vi "Check and Create Kalman Data.vi"(8 "Variance Memory":i32=1, 9 "R":T1, 10 "Pk":T1, 11 "x_k":T1) -> (1 "R out":T1, 2 "Pk out":T1, 3 "x_k out":T1)   [LabVIEW 2018]
uses:
  <vilib>/Analysis/Matrix/Datatypes/RealMatrix.ctl
  <vilib>/Analysis/Matrix/Numeric/Conversions/Array To Matrix - RA2.vi
  <vilib>/Analysis/7linalg.llb/Create Special Real Matrix.vi
  <vilib>/Analysis/Matrix/NI_Matrix.lvlib
  <vilib>/Analysis/NI_AALPro.lvlib
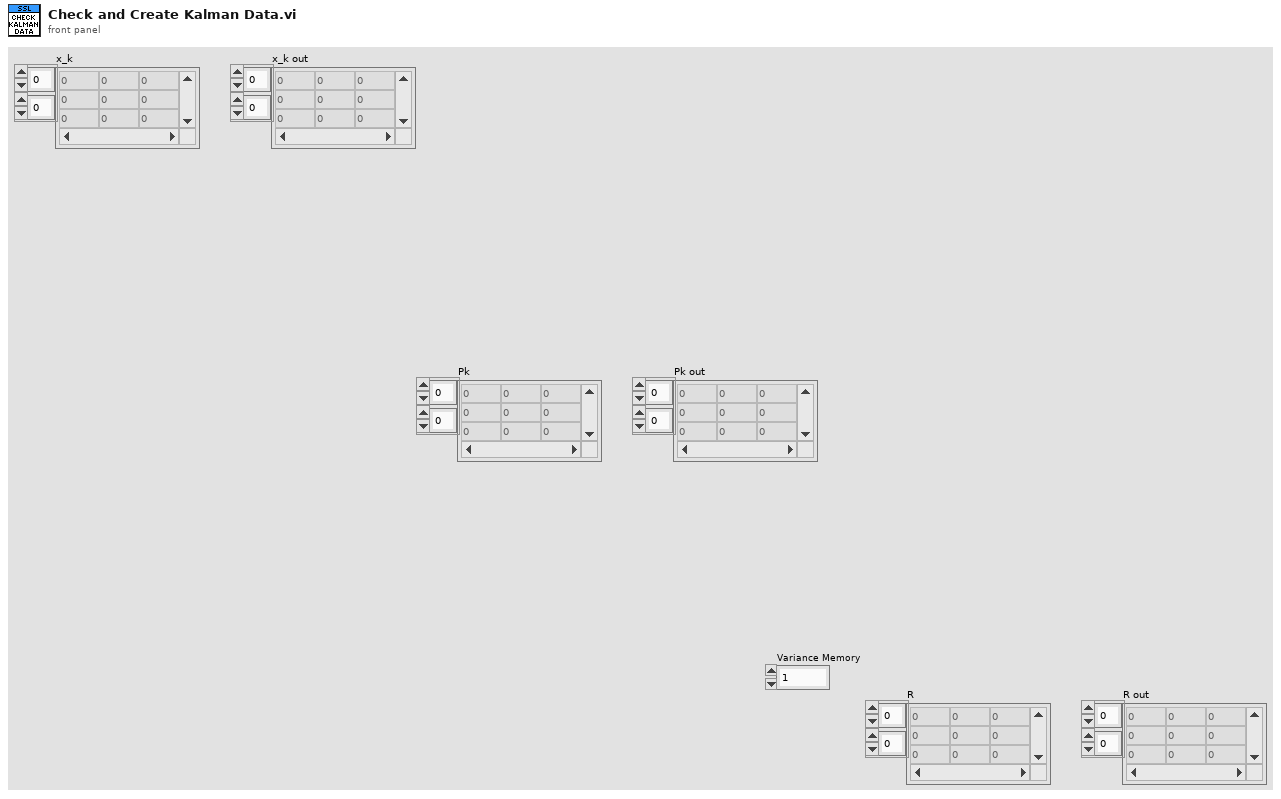
[diagram p1: front panel]
types:
  T1 = typedef "NI_Matrix.lvlib/RealMatrix.ctl" = dbl[][]
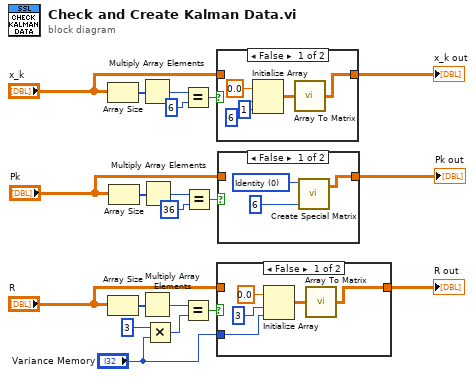
[diagram p0: block diagram]
diagram:
  n1 = Array Size(array="x_k") -> (size(s)=w15:i32[])
  n2 = Array Size(array="R") -> (size(s)=w4:i32[])
  n3 = Array Size(array="Pk") -> (size(s)=w9:i32[])
  n4 = Multiply Array Elements(1:w15) -> (0:w16:i32)
  n5 = Multiply Array Elements(1:w4) -> (0:w5:i32)
  n6 = Multiply Array Elements(1:w9) -> (0:w10:i32)
  n7 = Multiply(x=3, y="Variance Memory") -> (x*y=w3:i32)
  n8 = Equal?(x=w16, y=6) -> (x = y?=w18:bool)
  n9 = Equal?(x=w5, y=w3) -> (x = y?=w6:bool)
  n10 = Equal?(x=w10, y=36) -> (x = y?=w12:bool)
  n11 = case shown="False" w18 {
    tunnel: "x_k" -> [_ w26]
    tunnel: [w22 w26] -> w20
    frame False {
      n12 = Initialize Array(0.0 ("element"), 6 ("dimension size"), 1 ("dimension size")) -> (w23:dbl[][])
      n13 = call-poly <vilib>:"Array To Matrix.vi"("Real 2D Array"=w23) -> ("Real Matrix"=w22:T1)
    }
    frame True {
    }
  }
  "x_k out" <- w20
  n14 = case shown="False" w6 {
    tunnel: "R" -> [_ w32]
    tunnel: [w28 w32] -> w8
    tunnel: "Variance Memory" -> [w27 _]
    frame False {
      n15 = Initialize Array(0.0 ("element"), 3 ("dimension size"), w27) -> (w29:dbl[][])
      n16 = call-poly <vilib>:"Array To Matrix.vi"("Real 2D Array"=w29) -> ("Real Matrix"=w28:T1)
    }
    frame True {
    }
  }
  "R out" <- w8
  n17 = case shown="False" w12 {
    tunnel: "Pk" -> [_ w36]
    tunnel: [w33 w36] -> w14
    frame False {
      w35 = 0 items=["Identity", "Diagonal", "Toeplitz", "Vandermonde", "Companion", "Hankel", "Hadamard", "Wilkinson", "Hilbert", "Inverse Hilbert", "Rosser", "Pascal"] ("matrix type")
      n18 = call-poly <vilib>:"Create Special Matrix.vi"("matrix type"=w35, "matrix size"=6) -> ("Special Matrix"=w33:T1)  [unwired: 3 in, 1 out]
    }
    frame True {
    }
  }
  "Pk out" <- w14
